vi "CircleCalculations-Ver2-SubVI.vi"() -> ()   [LabVIEW 2018]
panel:
  in  "?":bool
  in  "?":bool
  out "Circumference":dbl format="%#_3g"
  out "Radius from Slider":dbl format="%#_2g"
  out "Area":dbl format="%#_4g"
  in  "Radius":dbl(slide) scale=0.0..10.0 scale format="%_2g"
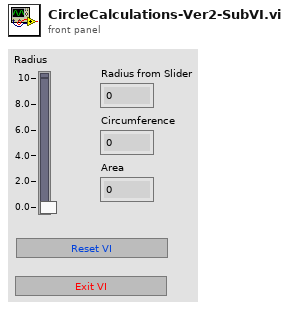
[diagram p1: front panel]
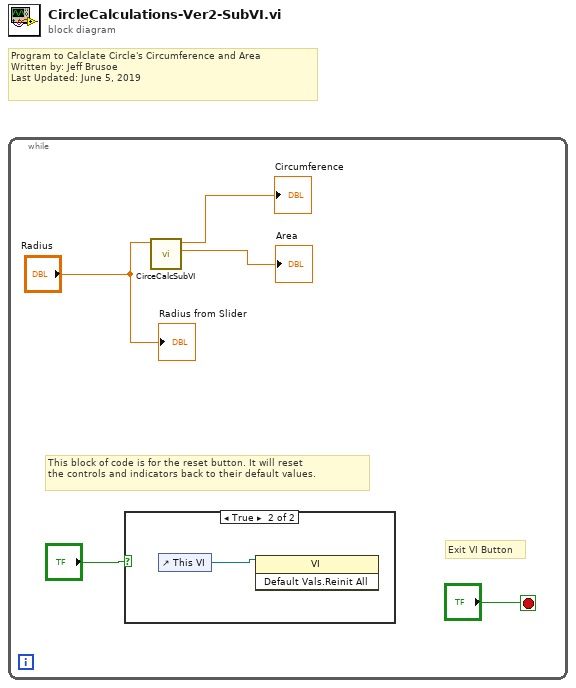
[diagram p0: block diagram]
diagram:
  # "Program to Calclate Circle's Circumference and Area\nWritten by: Jeff Brusoe\nLast Updated: June 5, 2019"
  n1 = while {
    stop <- "?" stop-if-true
    # "Exit VI Button"
    # "This block of code is for the reset button. It will reset\nthe controls and indicators back to their default values."
    n2 = case shown="True" "?" {
      frame False {
      }
      frame True {
        n3 = control-ref of="This VI"() -> (w6:refnum<vi>)
        n4 = invoke class="VI" method="Default Vals.Reinit All"(reference=w6) -> ()  [unwired: 2 in, 3 out]
      }
    }
    n5 = call "CirceCalcSubVI.vi"("Radius"="Radius") -> ("Numeric 2"=→"Area":dbl, "Numeric"=→"Circumference":dbl)  [unwired: 9 in]
    "Radius from Slider" <- "Radius"
  }
